vi "Deploy FPGATarget2.vi"(11 "session":u32) -> (3 "session out":u32)   [LabVIEW 2020, in "NI_TargetHelper.lvlib"]
uses:
  <vilib>/TargetSupport/NI_TargetHelper/NI_TargetHelper.lvlib
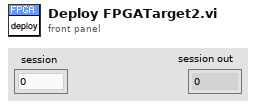
[diagram p1: front panel]
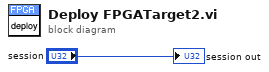
[diagram p0: block diagram]
diagram:
  "session out" <- "session"
